vi "SDT_GenerateInfoBlock.vi"(4 "ActiveModule":string[](array[string]), 6 "Contents":string="LV SDT-Data", 7 "FileType":T1=1 items=["non-Fifo"=1, "Fifo"=2, "FifoImage"=3], 9 "FileID":string="SPC FCS Data File", 10 "adc_re[exp]":i16=256, 11 "FilenameNoExtension":string) -> (3 "Info Block":string)   [LabVIEW 2017]
doc: "This VI is a SubVI to SDT_WriteFile.vi. and SPCWriteSETfoSPC.vi.\nIt formats the Info Block ready to be written to file. \nFor a description of the *.sdt file format see: SPC_data_file_structure.h\n\ninfo@becker-hickl.com"
uses:
  SPC_Wrappers/SPC_Controls/FileType.ctl
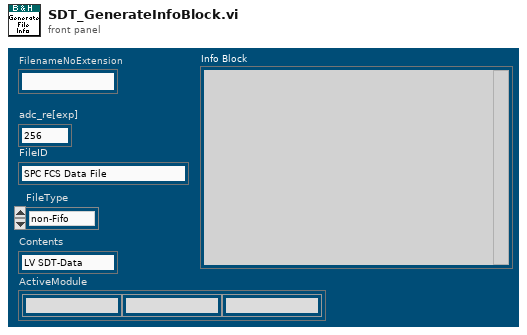
[diagram p1: front panel]
types:
  T1 = typedef "FileType.ctl" = u16
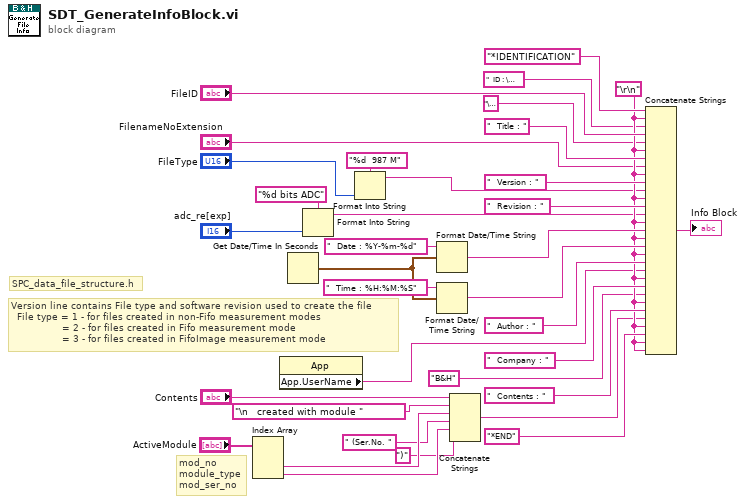
[diagram p0: block diagram]
diagram:
  w20 = "\r\n"
  # "mod_no\nmodule_type\nmod_ser_no"
  # "SPC_data_file_structure.h"
  # "Version line contains File type and software revision used to create the file \n  File type = 1 - for files created in non-Fifo measurement modes\n                 = 2 - for files created in Fifo measurement mode\n                 = 3 - for files created in FifoImage measurement mode"
  n1 = Index Array(array="ActiveModule") -> (element #2=w6:string, element #3=w4:string)  [unwired: 3 in, 1 out]
  n2 = property class="App"() -> ("App.UserName"=w2:string)  [unwired: 2 in, 2 out]
  n3 = Get Date/Time In Seconds() -> (seconds since 1Jan1904=w26:timestamp)
  n4 = Format Into String(format string="%d bits ADC", "adc_re[exp]") -> (resulting string=w17:string)  [unwired: 2 in, 1 out]
  n5 = Format Into String(format string="%d  987 M" ("Version"), "FileType") -> (resulting string=w10:string)  [unwired: 2 in, 1 out]
  n6 = Format Date/Time String(time format string (%c)="  Date : %Y-%m-%d", seconds (now)=w26) -> (date/time string=w29:string)  [unwired: 1 in]
  n7 = Format Date/Time String(time format string (%c)="  Time : %H:%M:%S", seconds (now)=w26) -> (date/time string=w27:string)  [unwired: 1 in]
  n8 = Concatenate Strings("Contents", "\n   created with module " ("string"), w6, " (Ser.No. " ("string"), w4, ")" ("string")) -> (w8:string)
  n9 = Concatenate Strings("*IDENTIFICATION", w20, "  ID : \u0004" ("FileID"), "FileID", "\u0004" ("string"), w20, "  Title : ", "FilenameNoExtension", w20, "  Version : ", w10, w20, "  Revision : ", w17, w20, w29, w20, w27, w20, "  Author : ", w2, w20, "  Company : ", "B&H" ("Company"), w20, "  Contents : ", w8, w20, "*END", w20, w20) -> (→"Info Block":string)
